vi "探头模板-12-网络版.vi"(11 "探头序号":T12(ring) caption="探头地址") -> ()   [LabVIEW 2017]
uses:
  <vilib>/Utility/miscctls.llb/LVPoint32TypeDef.ctl
  <vilib>/Utility/miscctls.llb/LVPositionTypeDef.ctl
  472b0359-2eb9-43bd-80a0-de906e95224b.vi
panel:
  out "初始尺寸":T1
  out "报警方式a":T2
  out "探头状态a":T3
  in  "报警方式[]":string[](array[string])
  out "累积":string="累积剂量/限值："
  in  "鼠标坐标":T4 caption="坐标"
  out "计算时间":dbl
  in  "坐标映射信号":bool=TRUE
  in  "探头属性":T5={"探头地址与信息"={"网络地址"="", "名称"="", "备注"="", "累积剂量"=0.0, "累积限值"=0.0, "硬件剂量率限值"=enum."一级限值", "剂量率限值1"=0.0, "剂量率限值2"=0.0, "报警方式"=enum."常报警"}, "测量值"={"时间"=timestamp(3554955153.6246996 s since 1904-01-01), "数值"=0.0}, "限值"={"限值1"=0.0, "限值2"=0.0, "探头限值"=enum."一级限值"}, "探头状态"=enum."正常", "累积记录"={"起始时间"=timestamp(0 s since 1904-01-01), "结束时间"=timestamp(0 s since 1904-01-01), "累积剂量"=0.0}, "报警方式"={"报警方式"=enum."常报警", "延迟计时"=0, "报警中？"=FALSE}}
  in  "停止":bool=TRUE
  out "探头地址":T12(ring)
  out "探头状态":enum16{"正常", "离线", "禁用", "一级报警", "二级报警", "累积报警"}(ring)=enum."一级报警"
  out "探头信息":string
  out "测量值":dbl format="%.2g"
  out "单位":enum16{"μ", "m"}(ring)
  out "限值1":string="一级限值："
  out "限值2":string="二级限值："
  out "数值":string="一级限值："
  in  "XY图":cluster{timestamp[], dbl[]}[](graph)
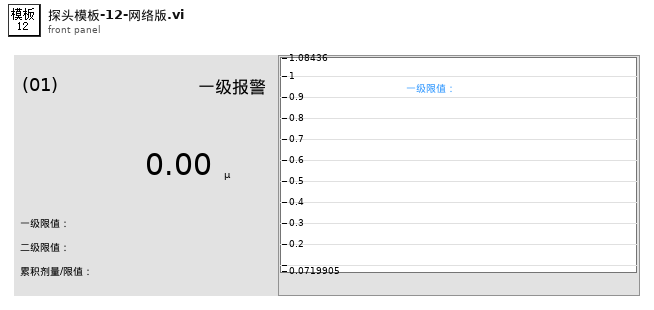
[diagram p1: front panel]
types:
  T1 = typedef "簇-界面模板初始字号.ctl" = cluster{"边界:区域高度":u32, "最大字号":cluster{"限值信息":u32, "测量值":u32, "序号":u32, "名称":u32, "单位":u32, "状态":u32, "悬浮框":u32}}
  T2 = typedef "报警方式选择.ctl" = enum16{"常报警", "自动静音", "手动静音"}
  T3 = typedef "探头状态.ctl" = enum16{"正常", "离线", "禁用", "一级报警", "二级报警", "累积报警"}
  T4 = typedef "LVPoint32TypeDef.ctl" = cluster{"Horizontal":i32, "Vertical":i32}
  T5 = typedef "探头属性.ctl" = cluster{"探头地址与信息":T6, "测量值":T8, "限值":T9, "探头状态":T3, "累积记录":T10, "报警方式":T11}
  T6 = typedef "探测器信息.ctl" = cluster{"网络地址":string, "名称":string, "备注":string, "累积剂量":dbl, "累积限值":dbl, "硬件剂量率限值":T7, "剂量率限值1":dbl, "剂量率限值2":dbl, "报警方式":T2}
  T7 = typedef "探头剂量率限值选择.ctl" = enum16{"一级限值", "二级限值"}
  T8 = typedef "测量值.ctl" = cluster{"时间":timestamp, "数值":dbl}
  T9 = typedef "剂量率限值.ctl" = cluster{"限值1":dbl, "限值2":dbl, "探头限值":T7}
  T10 = typedef "单条累积记录.ctl" = cluster{"起始时间":timestamp, "结束时间":timestamp, "累积剂量":dbl}
  T11 = typedef "报警方式.ctl" = cluster{"报警方式":T2, "延迟计时":u16, "报警中？":bool}
  T12 = enum16{"(01)", "(02)", "(03)", "(04)", "(05)", "(06)", "(07)", "(08)", "(09)", "(10)", "(11)", "(12)", "(13)", "(14)", "(15)", "(16)", "(17)", "(18)", "(19)", "(20)", "(21)", "(22)", "(23)", "(24)", "(25)", "(26)", "(27)", "(28)", "(29)", "(30)", "(31)", "(32)", "(33)", "(34)", "(35)"}
  T13 = cluster{"限值信息":u32, "测量值":u32, "序号":u32, "名称":u32, "单位":u32, "状态":u32, "悬浮框":u32}
  T14 = typedef "LVPositionTypeDef.ctl" = cluster{"Left":i32, "Top":i32}
  T15 = cluster{"原始尺寸":cluster{"所在窗格高度":u32, "字号":u32}, "new所在窗格高度":u32}
  T16 = enum16{"No Scaling", "Scale All Objects", "Scale Single Object"}
  T17 = typedef "LVBoundsTypeDef.ctl" = cluster{"Width":u32, "Height":u32}
  T18 = enum8{"Enabled", "Disabled", "Disabled and Grayed Out"}
  T19 = typedef "LVRectTypeDef.ctl" = cluster{"Left":i16, "Top":i16, "Right":i16, "Bottom":i16}
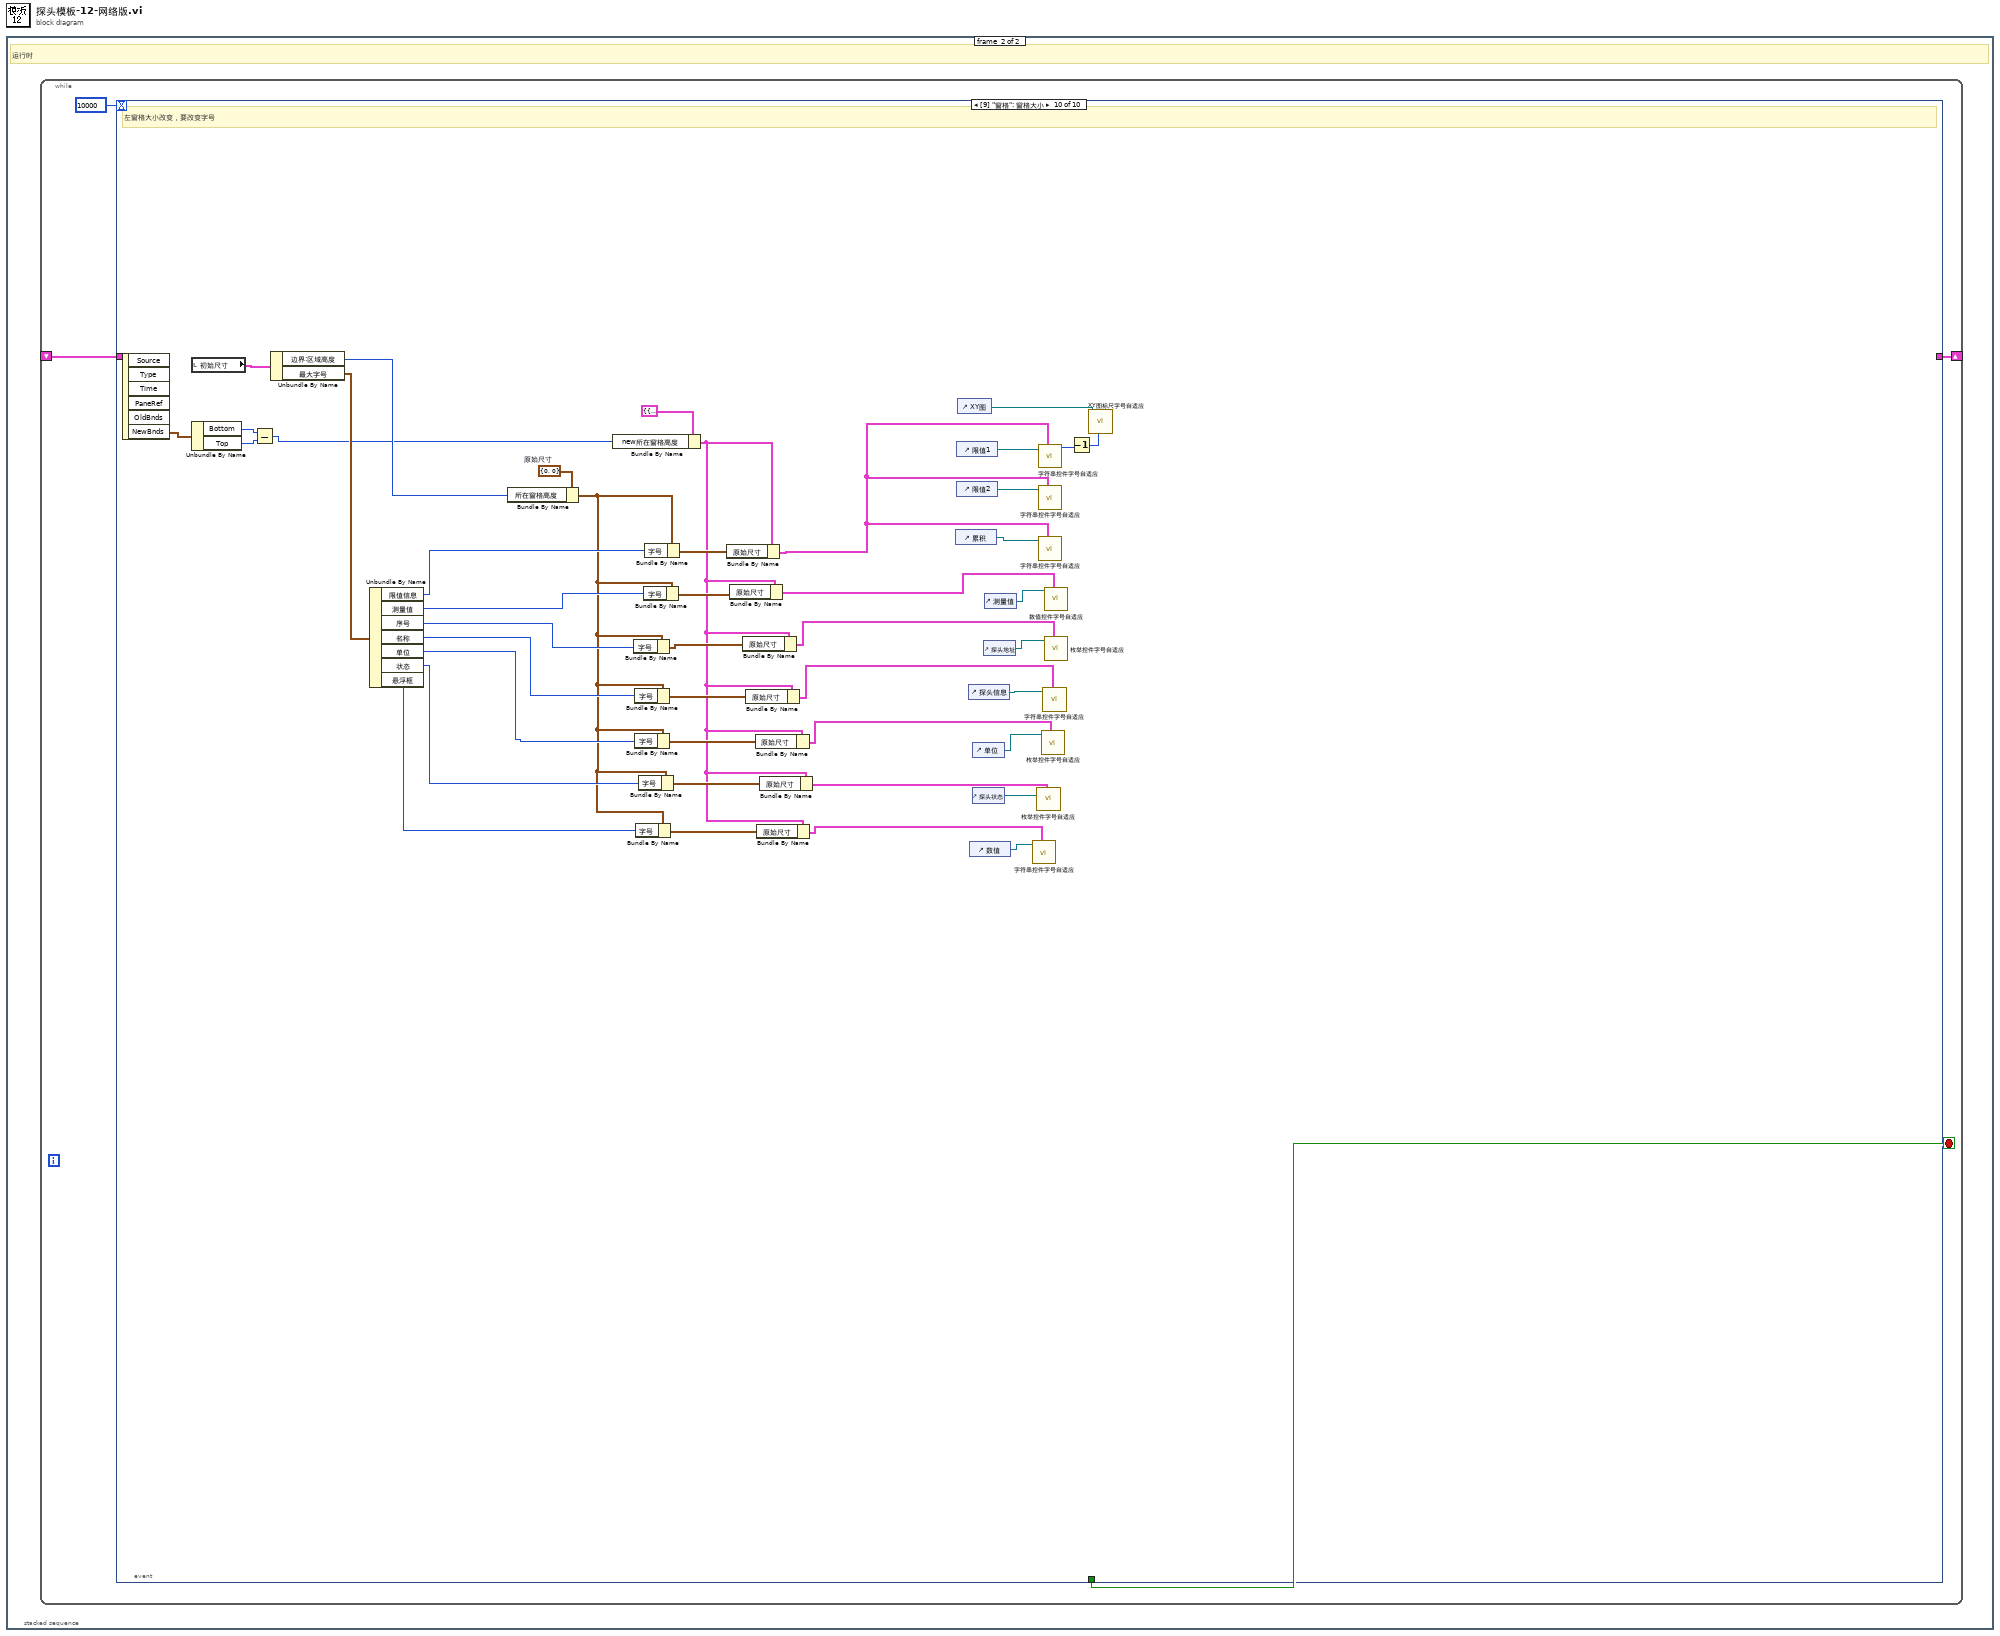
[diagram p0: block diagram]
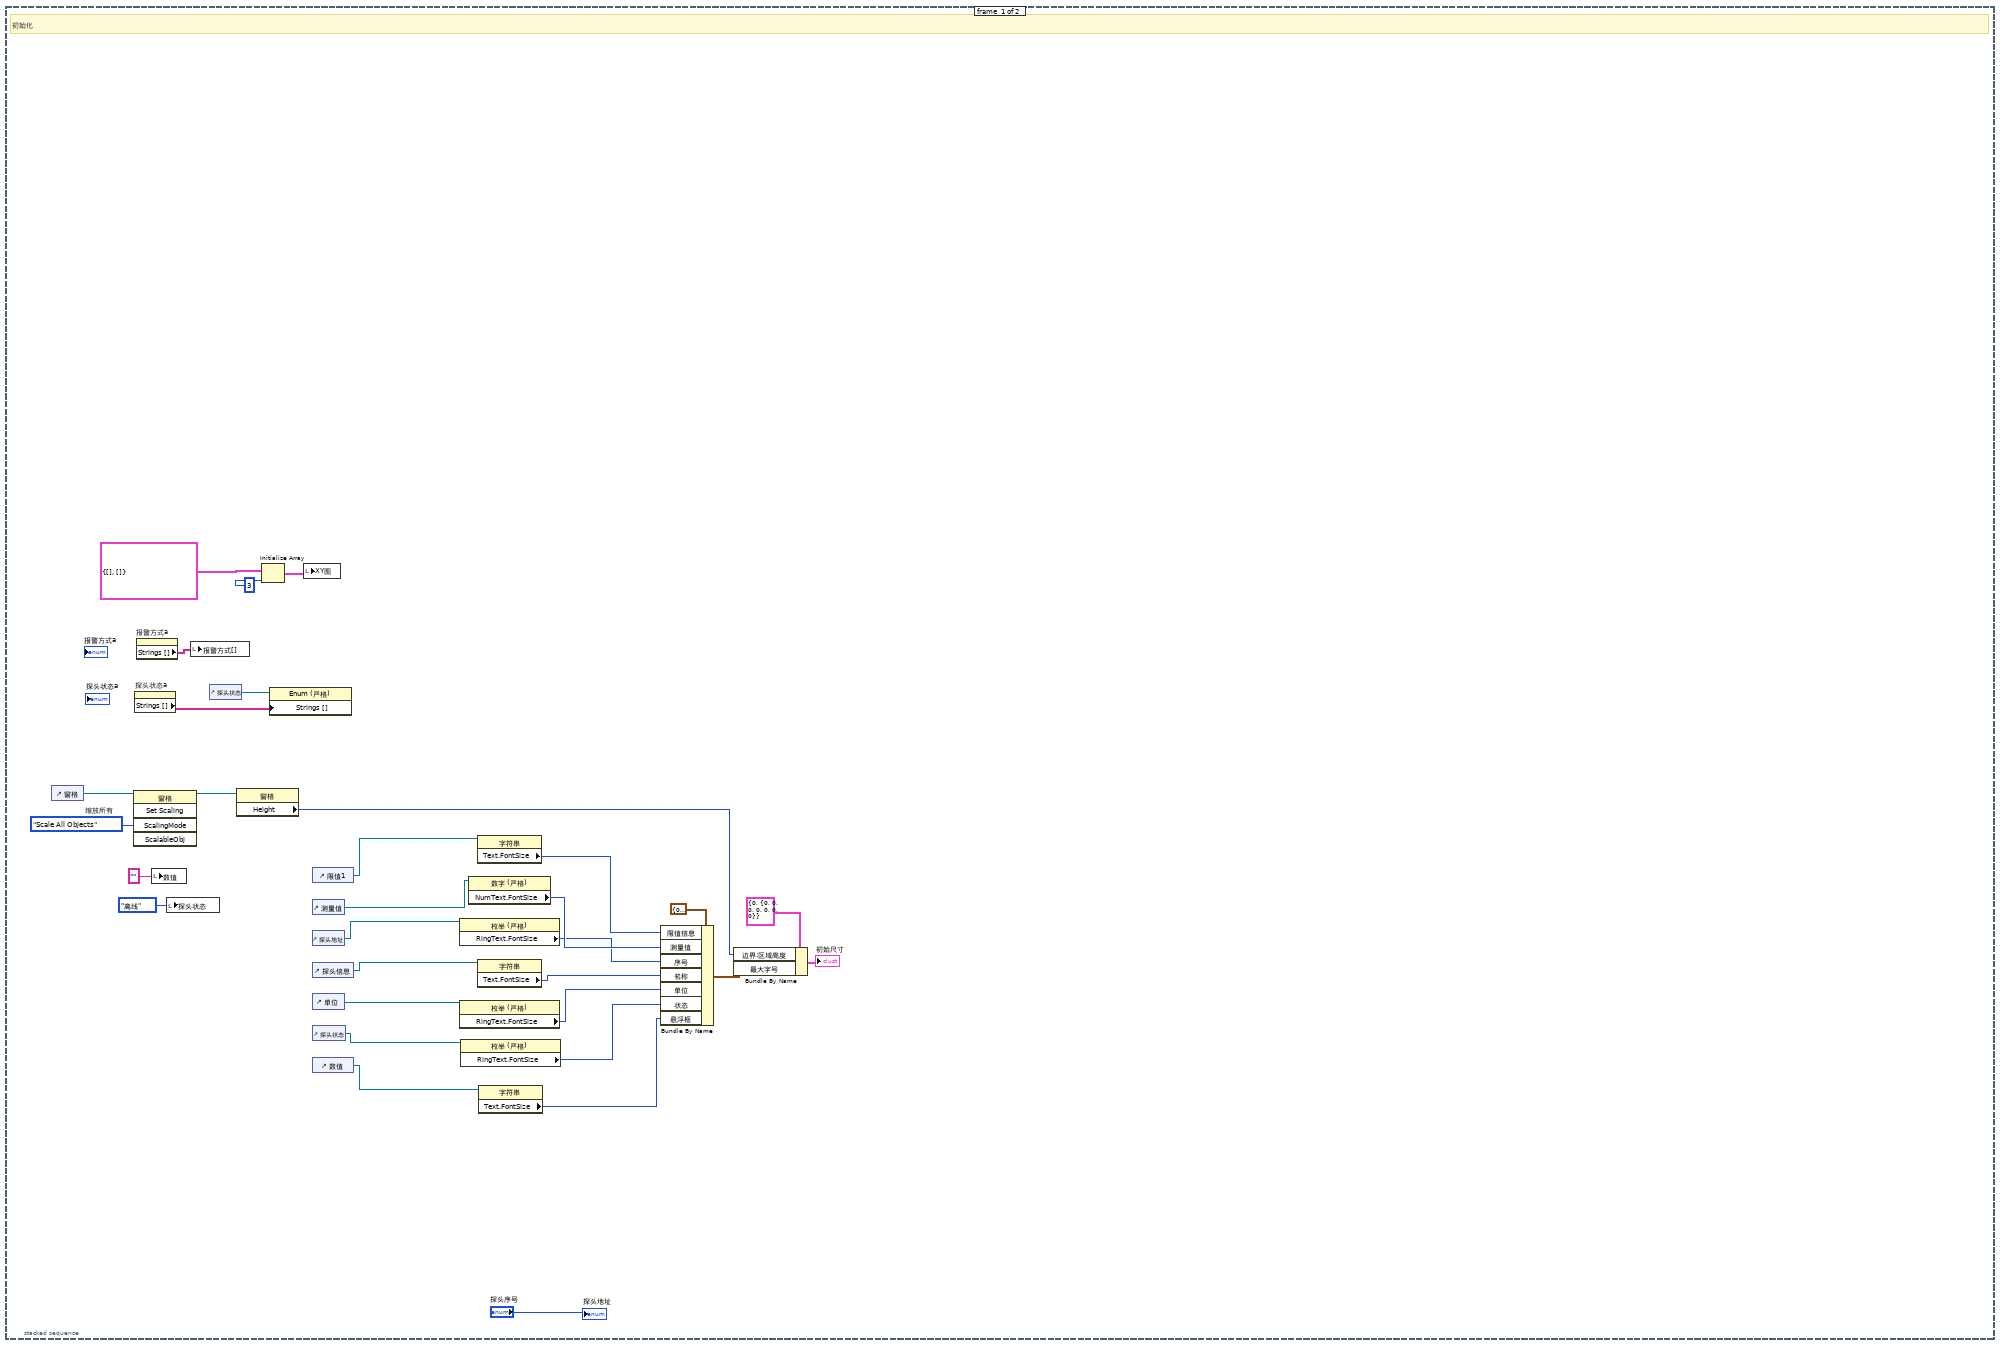
[diagram p2: hidden frame]
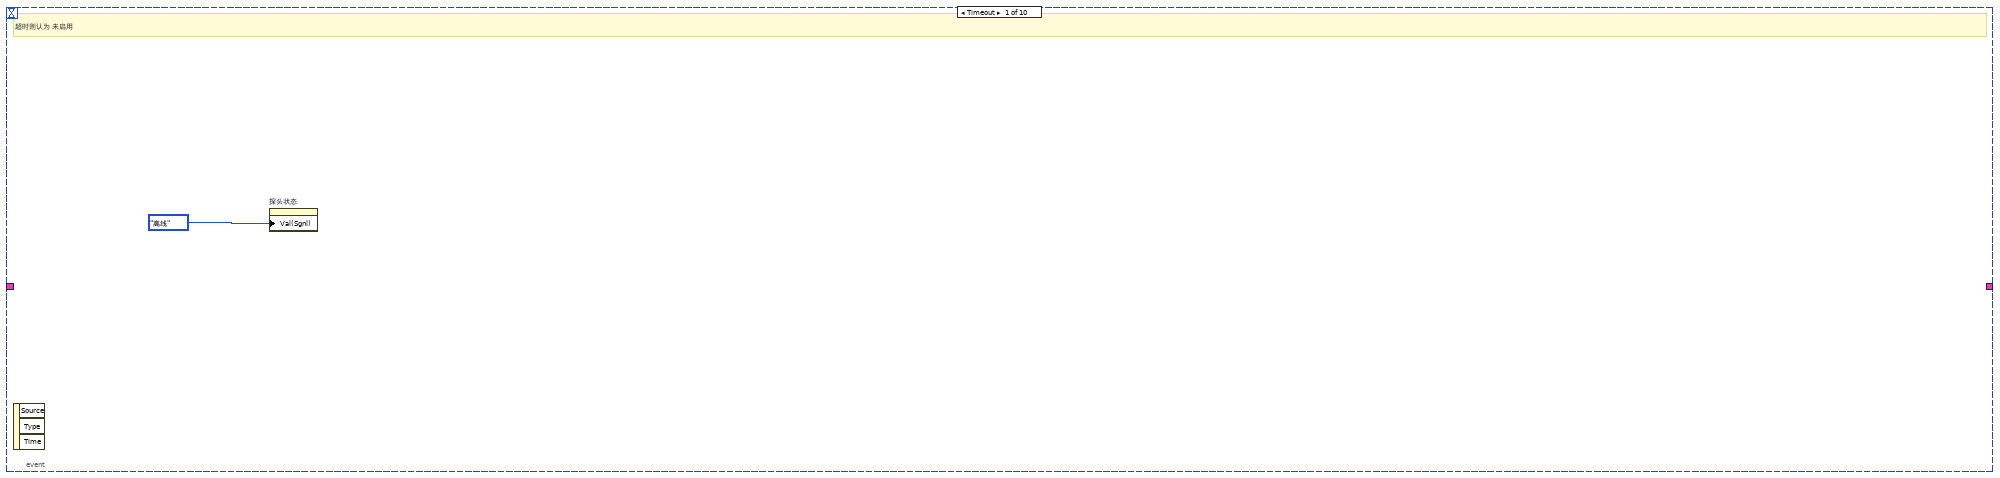
[diagram p3: hidden frame]
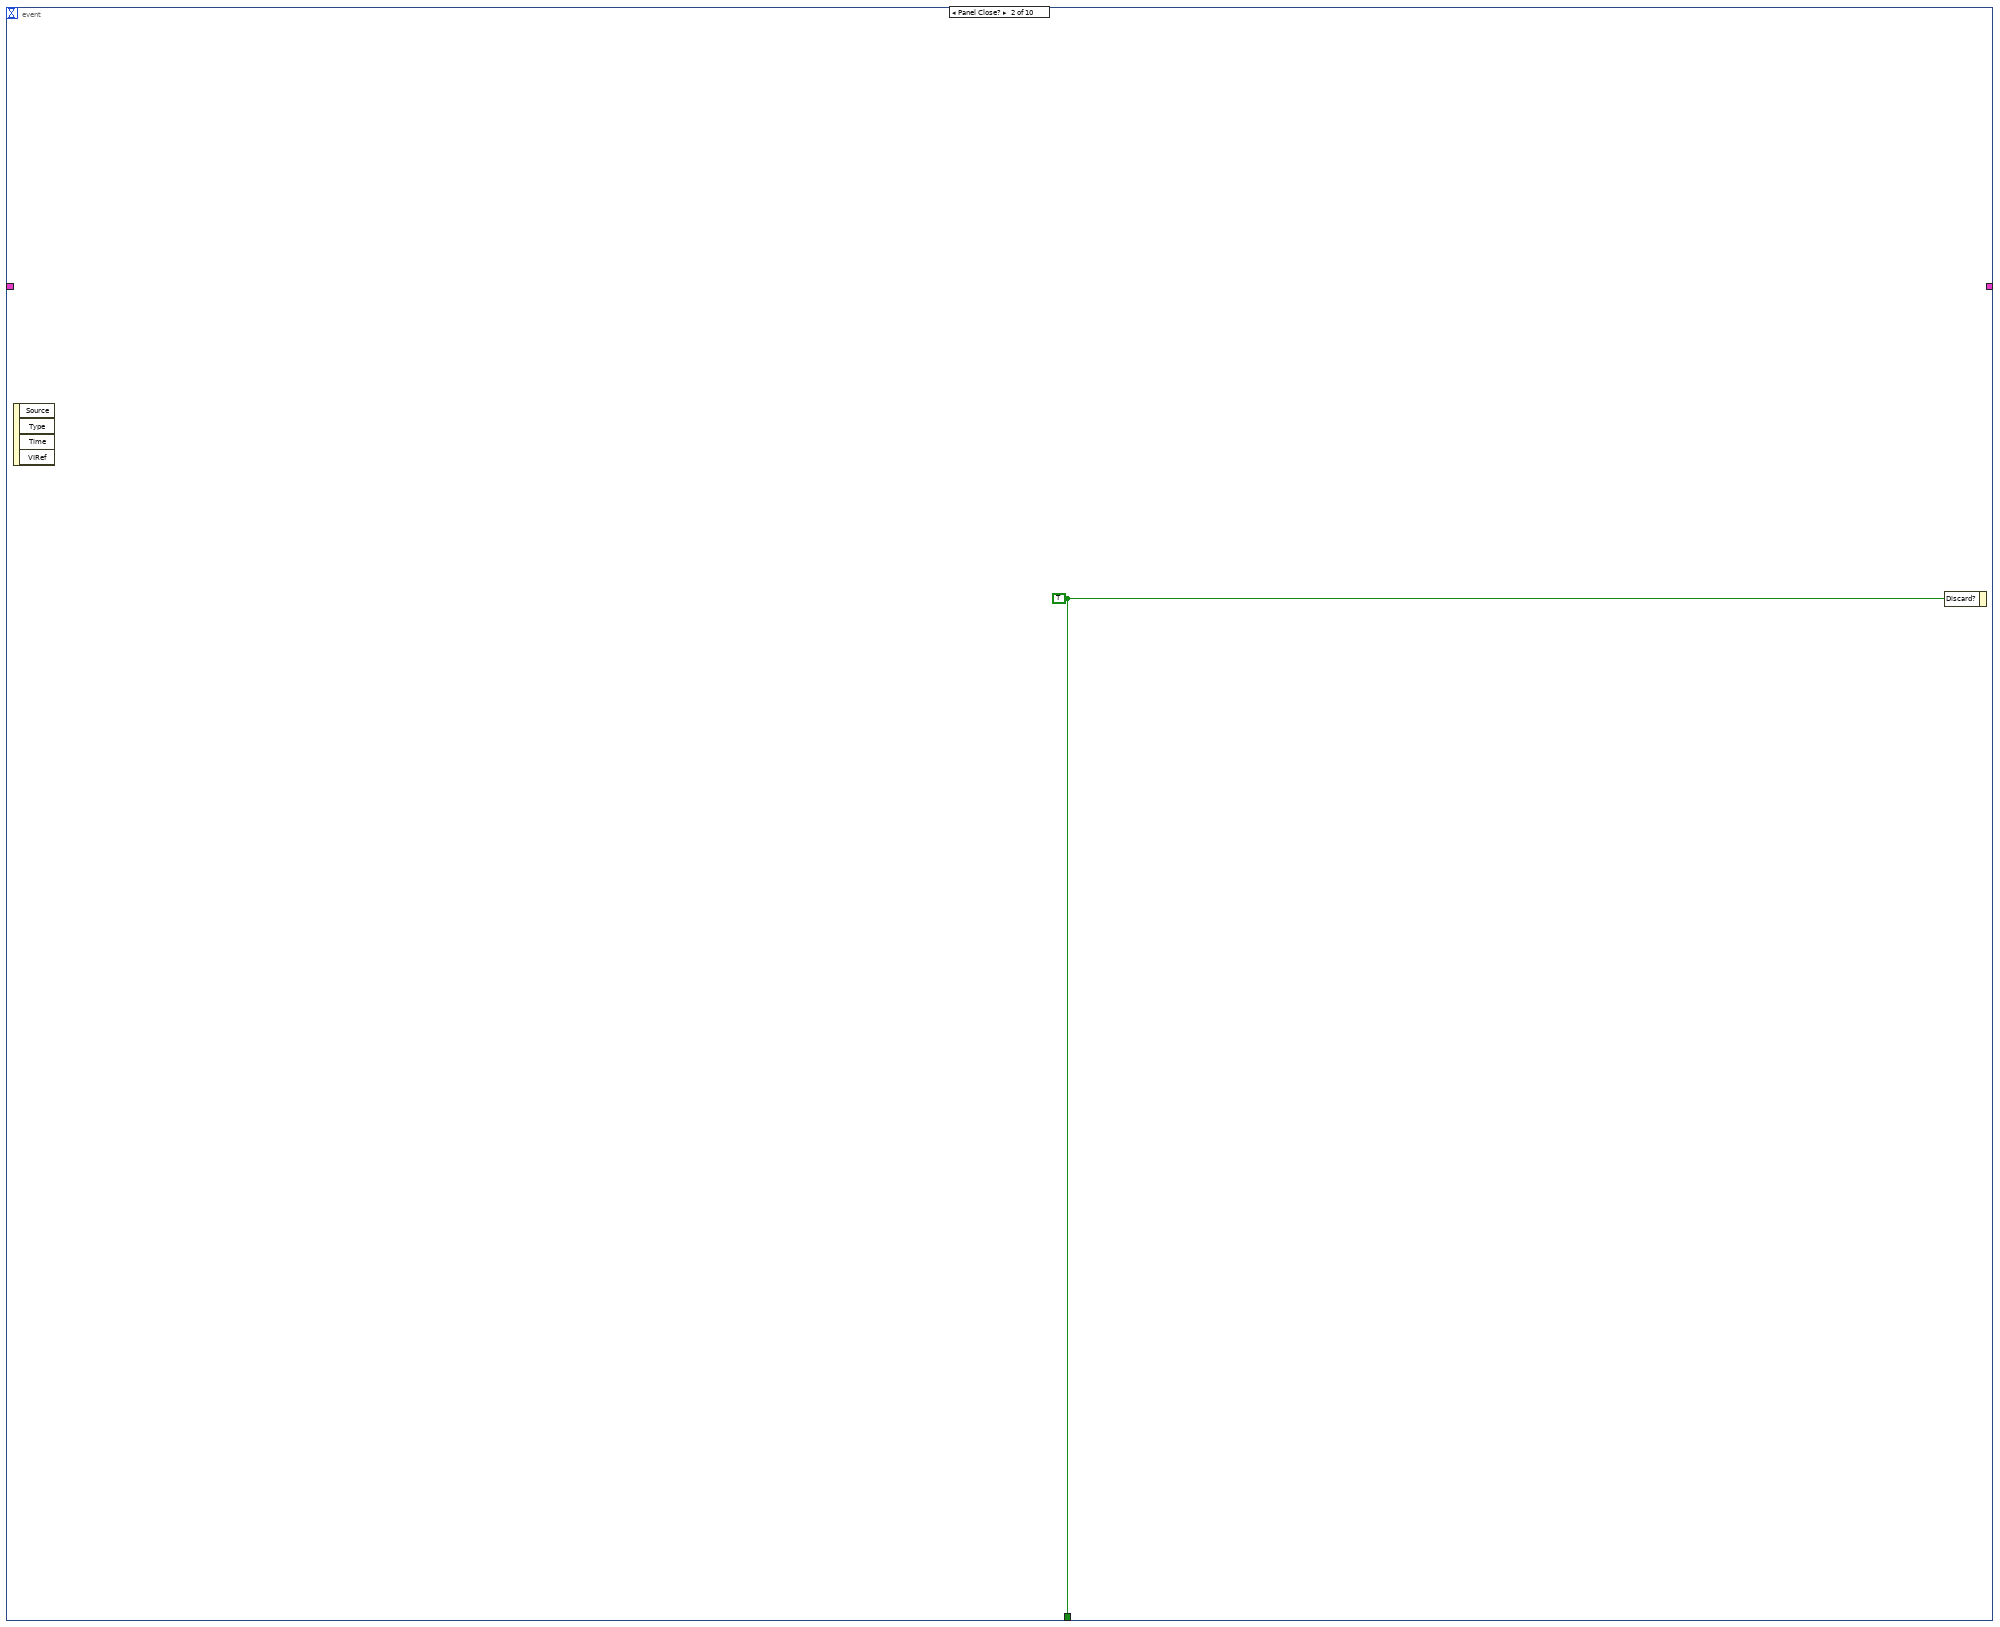
[diagram p4: hidden frame]
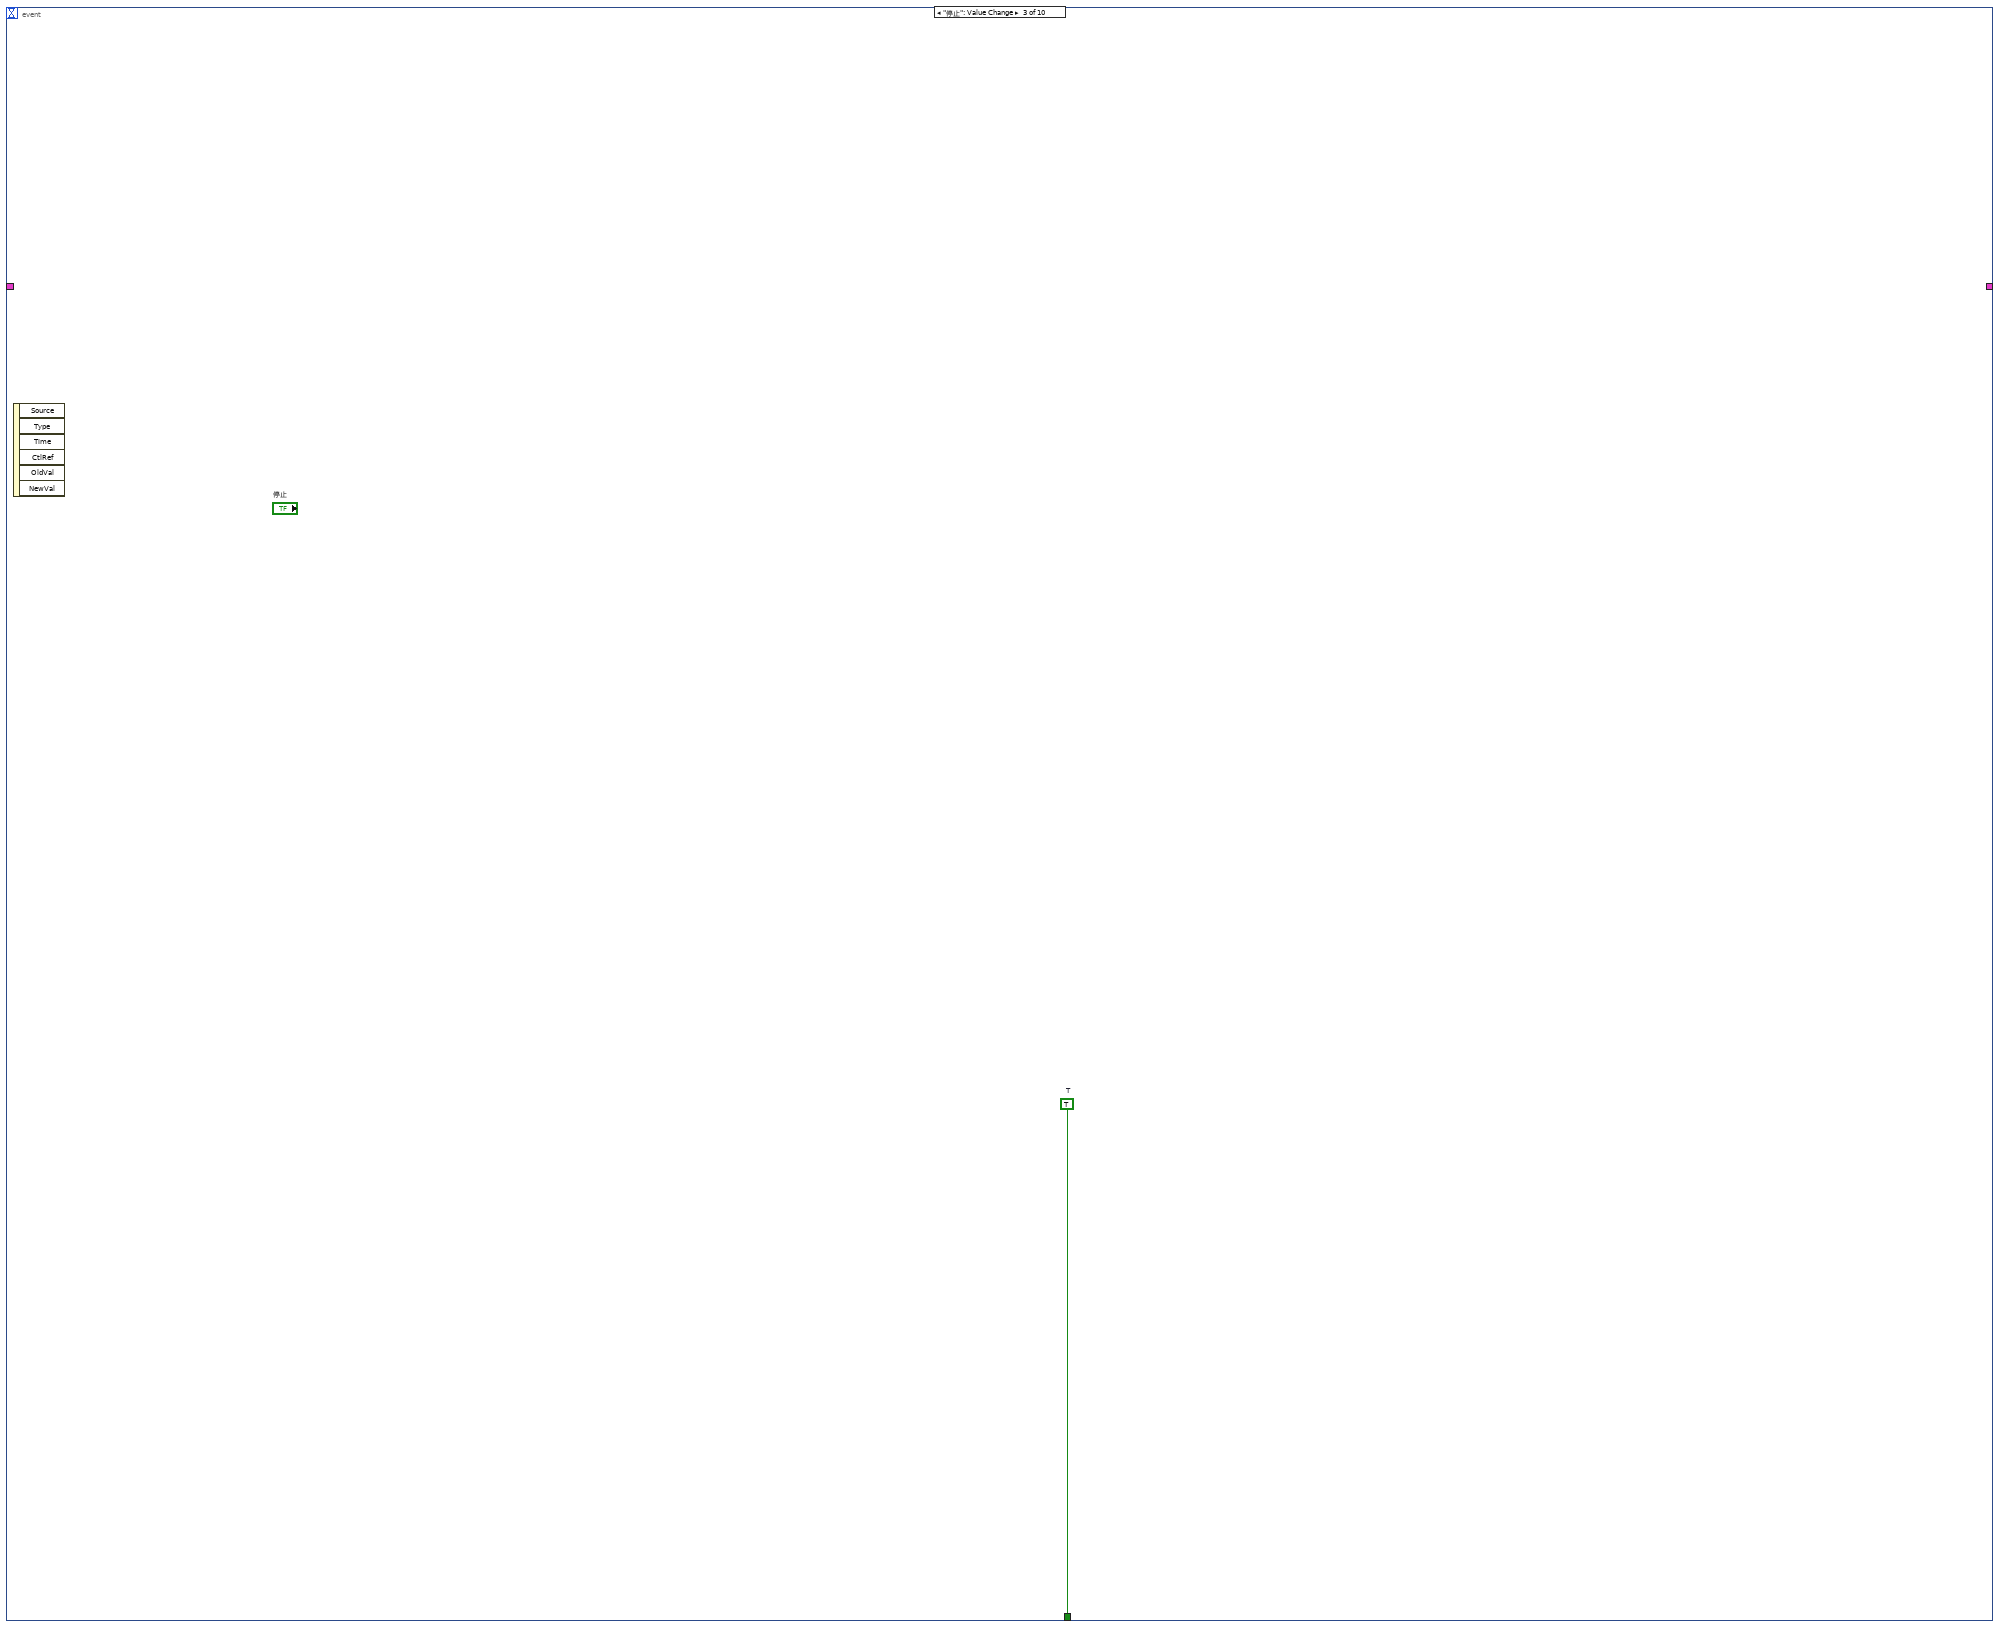
[diagram p5: hidden frame]
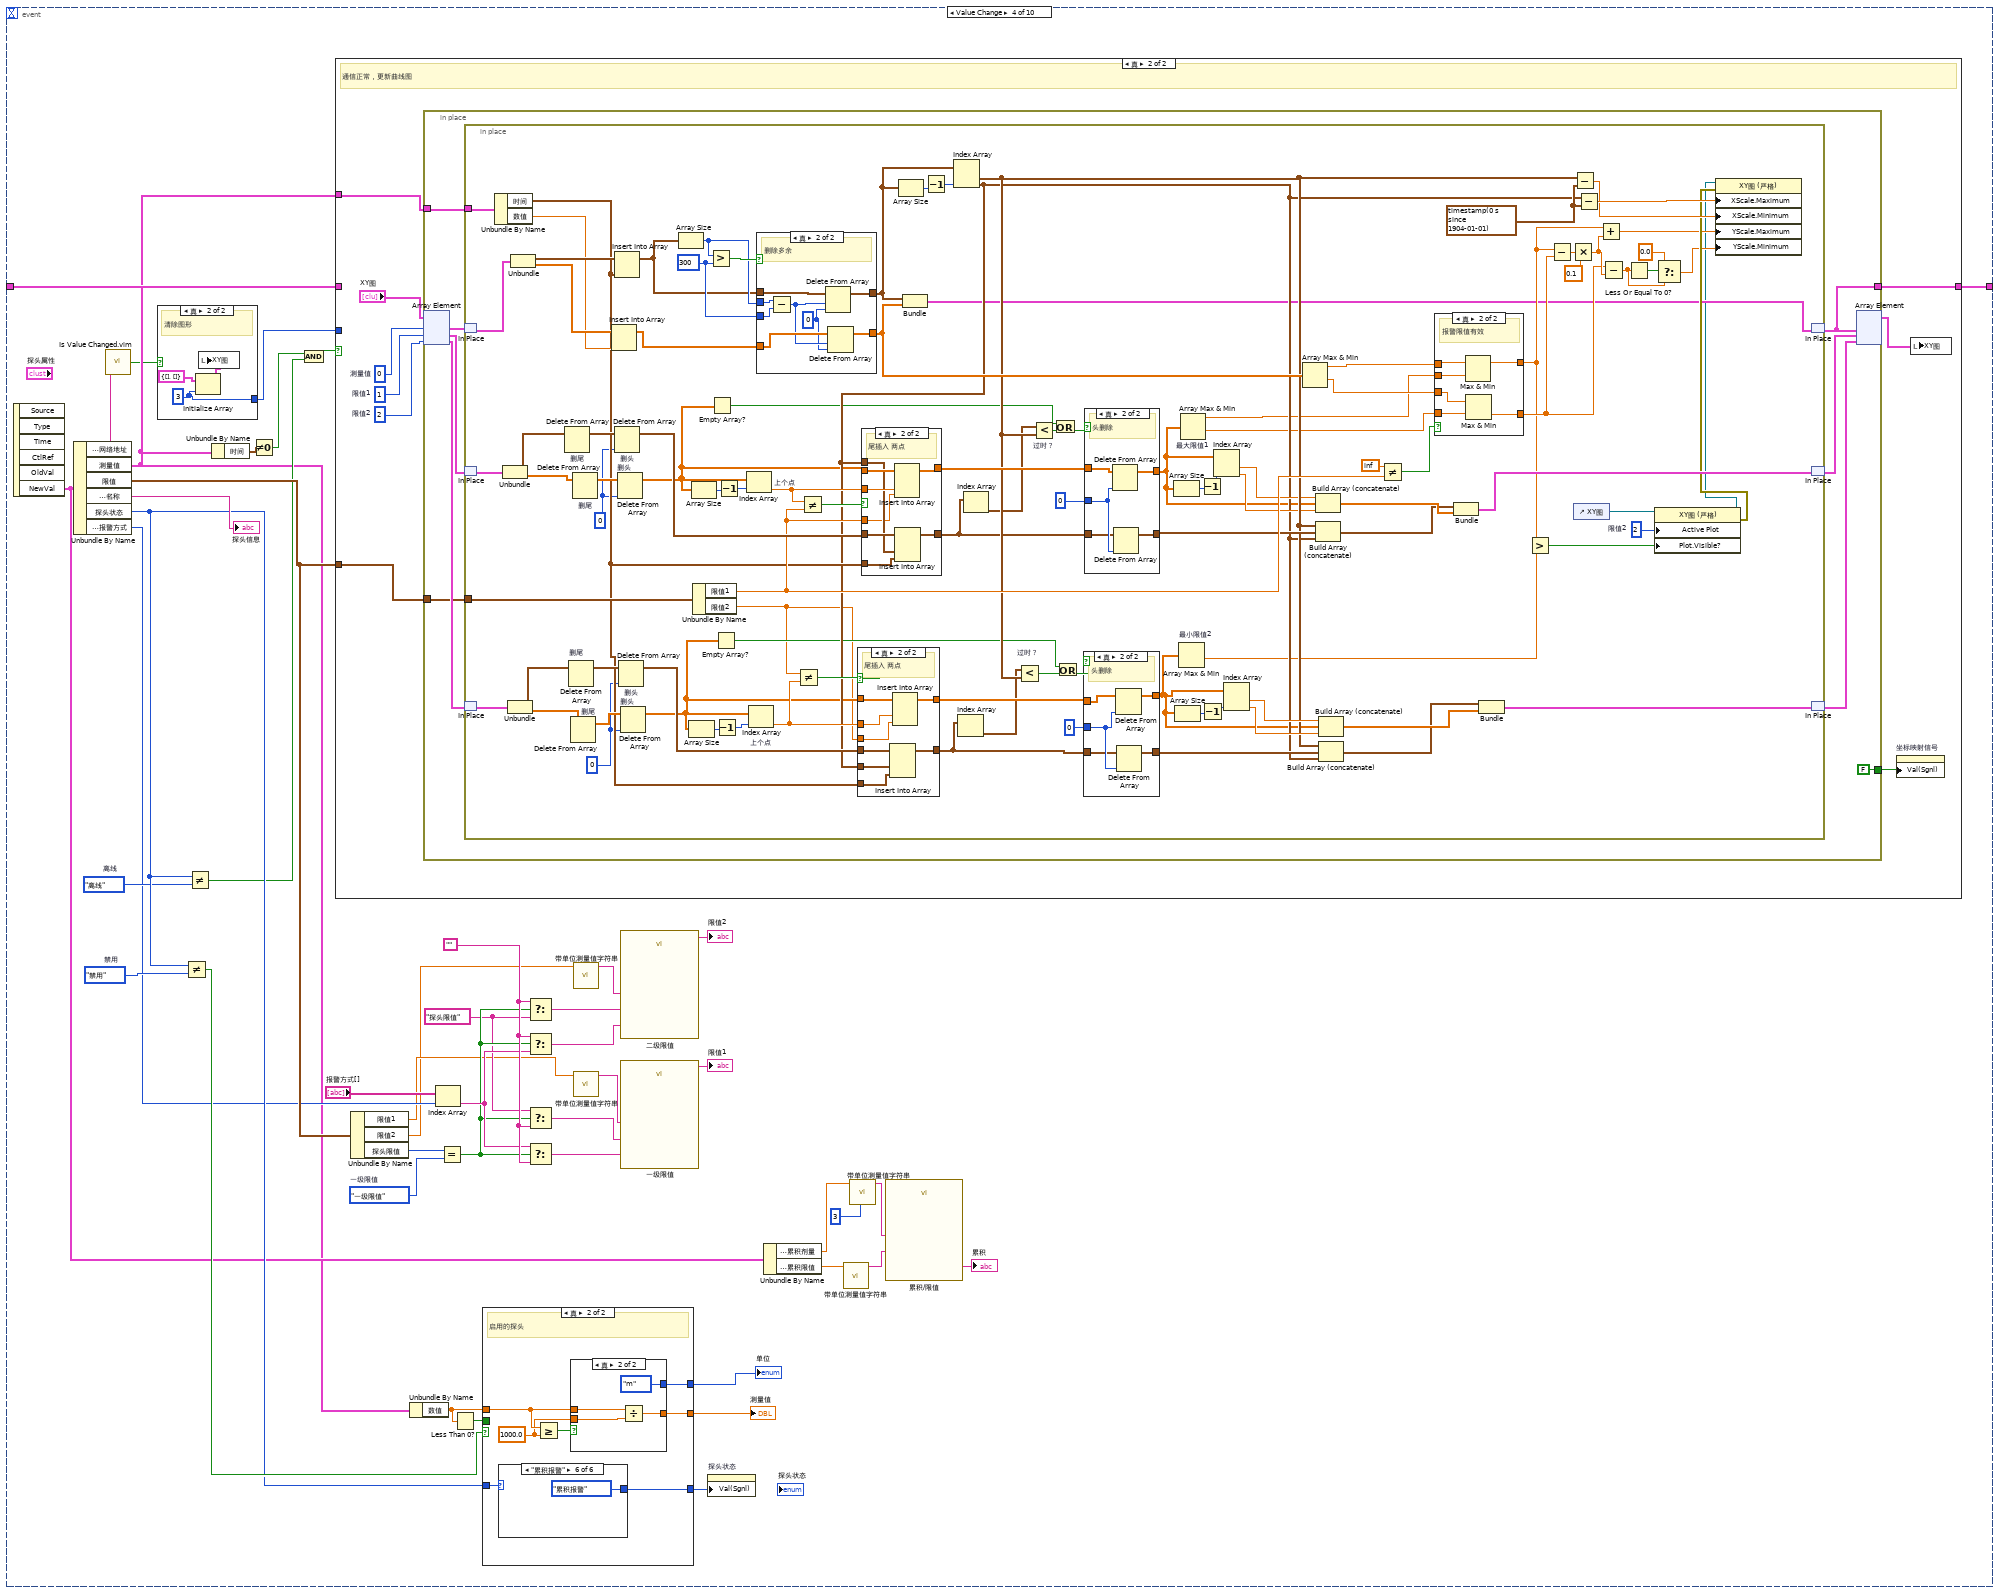
[diagram p6: hidden frame]
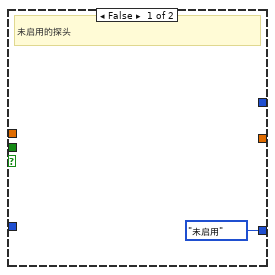
[diagram p15: hidden frame]
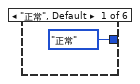
[diagram p16: hidden frame]
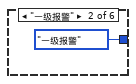
[diagram p17: hidden frame]
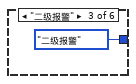
[diagram p18: hidden frame]
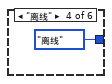
[diagram p19: hidden frame]
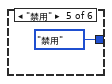
[diagram p20: hidden frame]
diagram:
  n1 = stacked-sequence {
    frame #0 {
      w24 = T16."Scale All Objects"  # 缩放所有
      # "初始化"
      n2 = control-ref of="窗格"() -> (w23:refnum<vi>)
      n3 = invoke class="窗格" method="Set Scaling"(reference=w23, "ScalingMode"=w24) -> (reference out=w20:refnum<vi>)  [unwired: 3 in, 4 out]
      n4 = property on="探头状态a" class="Enum (严格)"() -> ("Strings []"=w22:string[])  [unwired: 2 in, 2 out]
      n5 = property on="报警方式a" class="Enum (严格)"() -> ("Strings []"=w25:string[])  [unwired: 2 in, 2 out]
      n6 = local write "数值"("" ("数值")) -> ()
      n7 = local write "探头状态"(探头状态."离线" ("探头状态")) -> ()
      n8 = local write "报警方式[]"(w25) -> ()
      n9 = control-ref of="探头状态"() -> (w26:refnum<vi>)
      n10 = property class="窗格"(reference=w20) -> ("Height"=w1:u32)  [unwired: 1 in, 2 out]
      n11 = Initialize Array(cluster{timestamp[], dbl[]} {[], []}, 3 ("维数大小")) -> (w21:cluster{timestamp[], dbl[]}[])
      n12 = property on="属性节点" class="Enum (严格)"(reference=w26, "Strings []"=w22) -> ()  [unwired: 1 in, 2 out]
      n13 = local write "XY图"(w21) -> ()
      n14 = control-ref of="限值1"() -> (w15:refnum<vi>)
      n15 = control-ref of="测量值"() -> (w14:refnum<vi>)
      n16 = control-ref of="探头地址"() -> (w13:refnum<vi>)
      n17 = control-ref of="探头信息"() -> (w12:refnum<vi>)
      n18 = control-ref of="单位"() -> (w11:refnum<vi>)
      n19 = control-ref of="数值"() -> (w9:refnum<vi>)
      n20 = control-ref of="探头状态"() -> (w10:refnum<vi>)
      n21 = property class="枚举 (严格)"(reference=w13) -> ("RingText.FontSize"=w6:u32)  [unwired: 1 in, 2 out]
      n22 = property class="枚举 (严格)"(reference=w11) -> ("RingText.FontSize"=w4:u32)  [unwired: 1 in, 2 out]
      n23 = property class="枚举 (严格)"(reference=w10) -> ("RingText.FontSize"=w3:u32)  [unwired: 1 in, 2 out]
      n24 = property class="数字 (严格)"(reference=w14) -> ("NumText.FontSize"=w7:u32)  [unwired: 1 in, 2 out]
      n25 = property class="字符串"(reference=w15) -> ("Text.FontSize"=w8:u32)  [unwired: 1 in, 2 out]
      n26 = property class="字符串"(reference=w12) -> ("Text.FontSize"=w5:u32)  [unwired: 1 in, 2 out]
      n27 = property class="字符串"(reference=w9) -> ("Text.FontSize"=w2:u32)  [unwired: 1 in, 2 out]
      n28 = Bundle By Name(cluster=T13 {"限值信息"=0, "测量值"=0, "序号"=0, "名称"=0, "单位"=0, "状态"=0, "悬浮框"=0} ("最大字号"), "限值信息"=w8, "测量值"=w7, "序号"=w6, "名称"=w5, "单位"=w4, "状态"=w3, "悬浮框"=w2) -> (w19:T13)
      n29 = Bundle By Name(cluster=T1 {"边界:区域高度"=0, "最大字号"={"限值信息"=0, "测量值"=0, "序号"=0, "名称"=0, "单位"=0, "状态"=0, "悬浮框"=0}} ("输出簇"), "边界:区域高度"=w1, "最大字号"=w19) -> (→"初始尺寸":T1)
      "探头地址" <- "探头序号"
    }
    frame #1 {
      # "运行时"
      n30 = while {
        shift-right: [w34] -> _
        shift-left: _ -> [w33]
        stop <- w35 stop-if-true
        n31 = event shown="[9] \"窗格\": 窗格大小" {
          selector: _ -> [_ _ _ _ _ _ _ _ _ _]
          dyn-events: _ -> [_ _ _ _ _ _ _ _ _ _]
          timeout: 10000 -> [_ _ _ _ _ _ _ _ _ _]
          tunnel: [_ w37 w38 _ _ _ _ _ _ _] -> w35
          tunnel: [_ _ _ w72 w281 w283 w285 w290 w351 _] -> w34
          tunnel: w33 -> [_ _ _ w71 w281 w283 w285 w290 w351 _]
          event Timeout {
            # "超时则认为 未启用"
            n32 = event-data() -> ()  [unwired: 1 in, 3 out]
            n33 = property on="探头状态" class="Enum (严格)"("Val(Sgnl)"=探头状态."离线" ("值(信号)")) -> ()  [unwired: 2 in, 2 out]
          }
          event Panel Close? {
            w37 = TRUE ("放弃？")
            n34 = event-data() -> ()  [unwired: 1 in, 4 out]
            n35 = event-data("Discard?"=w37) -> ()  [unwired: 1 in, 1 out]
          }
          event "停止": Value Change {
            w38 = TRUE  # T
            n36 = event-data() -> ()  [unwired: 1 in, 6 out]
          }
          event Value Change {
            w70 = ""
            w67 = "探头限值" ("F-格式字符串")
            w66 = 探头剂量率限值选择."一级限值"  # 一级限值
            w74 = 探头状态."离线"  # 离线
            w79 = 探头状态."禁用"  # 禁用
            n37 = event-data() -> ("NewVal"=w63:T5)  [unwired: 1 in, 5 out]
            n38 = Unbundle By Name(w63) -> ("探头地址与信息.网络地址"=w41:string, "测量值"=w44:T8, "限值"=w78:T9, "探头地址与信息.名称"=→"探头信息":string, "探头状态"=w75:T3, "探头地址与信息.报警方式"=w64:T2)
            n39 = call "Is Value Changed.vim"("value"=w41) -> ("changed or first call?"=w40:bool)
            n40 = case shown="真" w40 {
              tunnel: [_ w85] -> w39
              frame False {
              }
              frame True {
                w85 = 3 ("维数大小")
                # "清除图形"
                n41 = Initialize Array(cluster{timestamp[], dbl[]} {[], []}, w85) -> (w86:cluster{timestamp[], dbl[]}[])
                n42 = local write "XY图"(w86) -> ()
              }
            }
            n43 = Not Equal?(x=w75, y=w79) -> (x != y?=w76:bool)
            n44 = Not Equal?(x=w75, y=w74) -> (x != y?=w73:bool)
            n45 = Unbundle By Name(w44) -> ("时间"=w43:timestamp)
            n46 = Not Equal To 0?(x=w43) -> (x != 0?=w42:bool)
            n47 = And(x=w42, y=w73) -> (x .and. y?=w45:bool)
            n48 = case shown="真" w45 {
              tunnel: w44 -> [_ w97]
              tunnel: w78 -> [_ w92]
              tunnel: [w88 w90] -> w72
              tunnel: w71 -> [w88 _]
              tunnel: w39 -> [_ _]
              frame False {
                # "离线，不更新"
              }
              frame True {
                w93 = 2  # 限值2
                w94 = 1  # 限值1
                w95 = 0  # 测量值
                # "通信正常，更新曲线图"
                n49 = in-place {
                  in-place-border: w97 -> [w106]
                  in-place-border: w92 -> [w102]
                  in-place-border: [w99] -> w90
                  in-place-border: [FALSE ("值(信号)")] -> w89
                  n50 = in-place-array #1("XY图", w95, w94, w93) -> (w105:cluster{timestamp[], dbl[]}, w103:cluster{timestamp[], dbl[]}, w104:cluster{timestamp[], dbl[]})
                  n51 = in-place {
                    in-place-border: w106 -> [w202]
                    in-place-border: w102 -> [w196]
                    w132 = 0 ("索引")
                    w133 = 0 ("索引")
                    w194 = u32 2  # 限值2
                    w203 = 300 ("y")
                    w208 = timestamp(0 s since 1904-01-01)
                    n52 = in-place-match #2(w105) -> (w197:cluster{timestamp[], dbl[]})
                    n53 = in-place-match #3(w103) -> (w162:cluster{timestamp[], dbl[]})
                    n54 = in-place-match #4(w104) -> (w143:cluster{timestamp[], dbl[]})
                    n55 = Unbundle By Name(w202) -> ("时间"=w142:timestamp, "数值"=w193:dbl)
                    n56 = Unbundle(w162) -> (w166:timestamp[], w165:dbl[])
                    n57 = Unbundle(w143) -> (w147:timestamp[], w146:dbl[])
                    n58 = Unbundle(w197) -> (w201:timestamp[], w200:dbl[])
                    n59 = Delete From Array "删尾"(array=w166) -> (array with subset deleted=w167:timestamp[])  [unwired: 2 in, 1 out]
                    n60 = Delete From Array "删尾"(array=w147) -> (array with subset deleted=w148:timestamp[])  [unwired: 2 in, 1 out]
                    n61 = Delete From Array "删尾"(array=w146) -> (array with subset deleted=w145:dbl[])  [unwired: 2 in, 1 out]
                    n62 = Delete From Array "删尾"(array=w165) -> (array with subset deleted=w164:dbl[])  [unwired: 2 in, 1 out]
                    n63 = Insert Into Array(array=w200, new element=w193) -> (w198:dbl[])  [unwired: 1 in]
                    n64 = Insert Into Array(array=w201, new element=w142) -> (w199:timestamp[])  [unwired: 1 in]
                    n65 = Delete From Array "删头"(array=w167, index=w133) -> (array with subset deleted=w170:timestamp[])  [unwired: 1 in, 1 out]
                    n66 = Delete From Array "删头"(array=w164, index=w133) -> (array with subset deleted=w121:dbl[])  [unwired: 1 in, 1 out]
                    n67 = Delete From Array "删头"(array=w148, index=w132) -> (array with subset deleted=w152:timestamp[])  [unwired: 1 in, 1 out]
                    n68 = Delete From Array "删头"(array=w145, index=w132) -> (array with subset deleted=w120:dbl[])  [unwired: 1 in, 1 out]
                    n69 = Array Size(array=w199) -> (size(s)=w204:i32)
                    n70 = Array Size(array=w120) -> (size(s)=w149:i32)
                    n71 = Array Size(array=w121) -> (size(s)=w163:i32)
                    n72 = Unbundle By Name(w196) -> ("限值1"=w161:dbl, "限值2"=w115:dbl)
                    n73 = Greater?(x=w204, y=w203) -> (0:w205:bool)
                    n74 = Empty Array?(array=w121) -> (empty?=w119:bool)
                    n75 = Empty Array?(array=w120) -> (empty?=w118:bool)
                    n76 = Decrement(x=w149) -> (x-1=w150:i32)
                    n77 = Decrement(x=w163) -> (x-1=w168:i32)
                    n78 = Index Array "上个点"(array=w121, index=w168) -> (element=w131:dbl)
                    n79 = Index Array "上个点"(array=w120, index=w150) -> (element=w130:dbl)
                    n80 = case shown="真" w205 {
                      tunnel: w199 -> [w252 w260]
                      tunnel: w204 -> [_ w259]
                      tunnel: w203 -> [_ w258]
                      tunnel: [w252 w257] -> w192
                      tunnel: w198 -> [w251 w256]
                      tunnel: [w251 w253] -> w188
                      frame False {
                      }
                      frame True {
                        w254 = 0 ("索引")
                        # "删除多余"
                        n81 = Subtract(x=w259, y=w258) -> (x-y=w255:i32)
                        n82 = Delete From Array(array=w260, length=w255, index=w254) -> (array with subset deleted=w257:timestamp[])  [unwired: 1 out]
                        n83 = Delete From Array(array=w256, length=w255, index=w254) -> (array with subset deleted=w253:dbl[])  [unwired: 1 out]
                      }
                    }
                    n84 = Not Equal?(x=w115, y=w130) -> (x != y?=w144:bool)
                    n85 = Not Equal?(x=w131, y=w161) -> (x != y?=w134:bool)
                    n86 = Array Size(array=w192) -> (size(s)=w191:i32)
                    n87 = Bundle(w192, w188) -> (w109:cluster{timestamp[], dbl[]})  [unwired: 1 in]
                    n88 = Decrement(x=w191) -> (x-1=w190:i32)
                    n89 = Index Array(array=w192, index #2=w190) -> (element #1=w139:timestamp, element #2=w129:timestamp)  [unwired: 1 in]
                    n90 = case shown="真" w144 {
                      tunnel: [w217 w219] -> w128
                      tunnel: w120 -> [w217 w225]
                      tunnel: w115 -> [_ w218]
                      tunnel: w152 -> [w216 w224]
                      tunnel: w142 -> [_ w221]
                      tunnel: [w216 w220] -> w125
                      tunnel: w130 -> [_ w223]
                      tunnel: w129 -> [_ w222]
                      frame False {
                        # "不插入"
                      }
                      frame True {
                        # "尾插入 两点"
                        n91 = Insert Into Array(array=w224, new element #1=w222, new element #2=w221) -> (w220:timestamp[])  [unwired: 1 in]
                        n92 = Insert Into Array(array=w225, new element #1=w223, new element #2=w218) -> (w219:dbl[])  [unwired: 1 in]
                      }
                    }
                    n93 = case shown="真" w134 {
                      tunnel: [w234 w238] -> w171
                      tunnel: w121 -> [w234 w242]
                      tunnel: w161 -> [_ w235]
                      tunnel: w142 -> [_ w236]
                      tunnel: w170 -> [w233 w241]
                      tunnel: [w233 w237] -> w127
                      tunnel: w131 -> [_ w240]
                      tunnel: w129 -> [_ w239]
                      frame False {
                        # "不插入"
                      }
                      frame True {
                        # "尾插入 两点"
                        n94 = Insert Into Array(array=w242, new element #1=w240, new element #2=w235) -> (w238:dbl[])  [unwired: 1 in]
                        n95 = Insert Into Array(array=w241, new element #1=w239, new element #2=w236) -> (w237:timestamp[])  [unwired: 1 in]
                      }
                    }
                    n96 = Index Array(array=w125) -> (element=w124:timestamp)  [unwired: 1 in]
                    n97 = Index Array(array=w127) -> (element=w126:timestamp)  [unwired: 1 in]
                    n98 = Less? "过时？"(x=w124, y=w139) -> (x < y?=w151:bool)
                    n99 = Less? "过时？"(x=w126, y=w139) -> (x < y?=w169:bool)
                    n100 = Or(x=w119, y=w169) -> (x .or. y?=w123:bool)
                    n101 = Or(x=w118, y=w151) -> (x .or. y?=w122:bool)
                    n102 = case shown="真" w122 {
                      tunnel: w128 -> [w210 w214]
                      tunnel: w125 -> [w209 w213]
                      tunnel: 0 ("索引") -> [_ w215]
                      tunnel: [w210 w212] -> w117
                      tunnel: [w209 w211] -> w156
                      frame False {
                      }
                      frame True {
                        # "头删除"
                        n103 = Delete From Array(array=w214, index=w215) -> (array with subset deleted=w212:dbl[])  [unwired: 1 in, 1 out]
                        n104 = Delete From Array(array=w213, index=w215) -> (array with subset deleted=w211:timestamp[])  [unwired: 1 in, 1 out]
                      }
                    }
                    n105 = case shown="真" w123 {
                      tunnel: w171 -> [w227 w232]
                      tunnel: w127 -> [w226 w230]
                      tunnel: 0 ("索引") -> [_ w231]
                      tunnel: [w227 w229] -> w116
                      tunnel: [w226 w228] -> w140
                      frame False {
                      }
                      frame True {
                        # "头删除"
                        n106 = Delete From Array(array=w232, index=w231) -> (array with subset deleted=w229:dbl[])  [unwired: 1 in, 1 out]
                        n107 = Delete From Array(array=w230, index=w231) -> (array with subset deleted=w228:timestamp[])  [unwired: 1 in, 1 out]
                      }
                    }
                    n108 = Array Size(array=w116) -> (size(s)=w173:i32)
                    n109 = Array Size(array=w117) -> (size(s)=w155:i32)
                    n110 = Array Max & Min "最小限值2"(array=w117) -> (min value=w111:dbl)  [unwired: 3 out]
                    n111 = Array Max & Min "最大限值1"(array=w116) -> (max value=w114:dbl, min value=w113:dbl)  [unwired: 2 out]
                    n112 = Decrement(x=w173) -> (x-1=w174:i32)
                    n113 = Decrement(x=w155) -> (x-1=w154:i32)
                    n114 = Index Array(array=w116, index #2=w174) -> (element #1=w138:dbl, element #2=w137:dbl)  [unwired: 1 in]
                    n115 = Index Array(array=w117, index #2=w154) -> (element #1=w157:dbl, element #2=w158:dbl)  [unwired: 1 in]
                    n116 = Array Max & Min(array=w188) -> (max value=w179:dbl, min value=w178:dbl)  [unwired: 2 out]
                    n117 = Build Array (concatenate)(w138, w116, w137) -> (w136:dbl[])
                    n118 = Build Array (concatenate)(w139, w140, w129) -> (w135:timestamp[])
                    n119 = Build Array (concatenate)(w157, w117, w158) -> (w160:dbl[])
                    n120 = Build Array (concatenate)(w139, w156, w129) -> (w159:timestamp[])
                    n121 = Not Equal?(x=inf, y=w161) -> (x != y?=w176:bool)
                    n122 = case shown="真" w176 {
                      tunnel: w179 -> [w244 w250]
                      tunnel: [w244 w249] -> w112
                      tunnel: w113 -> [_ w248]
                      tunnel: w178 -> [w243 w247]
                      tunnel: [w243 w246] -> w177
                      tunnel: w114 -> [_ w245]
                      frame False {
                        # "报警限值 Inf 无效"
                      }
                      frame True {
                        # "报警限值有效"
                        n123 = Max & Min(x=w250, y=w245) -> (max(x,y)=w249:dbl)  [unwired: 1 out]
                        n124 = Max & Min(x=w247, y=w248) -> (min(x,y)=w246:dbl)  [unwired: 1 out]
                      }
                    }
                    n125 = Bundle(w135, w136) -> (w195:cluster{timestamp[], dbl[]})  [unwired: 1 in]
                    n126 = Bundle(w159, w160) -> (w141:cluster{timestamp[], dbl[]})  [unwired: 1 in]
                    n127 = Greater?(x=w112, y=w111) -> (0:w110:bool)
                    n128 = Subtract(x=w112, y=w177) -> (x-y=w187:dbl)
                    n129 = Multiply(x=w187, y=0.1) -> (x*y=w184:dbl)
                    n130 = Subtract(x=w139, y=w208) -> (x-y=w206:dbl)
                    n131 = control-ref of="XY图"() -> (w108:refnum<vi>)
                    n132 = Subtract(x=w129, y=w208) -> (x-y=w207:dbl)
                    n133 = Add(x=w112, y=w184) -> (x+y=w185:dbl)
                    n134 = Subtract(x=w177, y=w184) -> (x-y=w180:dbl)
                    n135 = Less Or Equal To 0?(x=w180) -> (x <= 0?=w183:bool)
                    n136 = property on="属性节点" class="XY图 (严格)"(reference=w108, "Active Plot"=w194, "Plot.Visible?"=w110) -> (reference out=w107:refnum<vi>, error out=w189:errorcluster)  [unwired: 1 in]
                    n137 = Select(t=0.0, s=w183, f=w180) -> (s? t:f=w181:dbl)
                    n138 = property on="属性节点" class="XY图 (严格)"(reference=w107, error in=w189, "XScale.Maximum"=w207, "XScale.Minimum"=w206, "YScale.Maximum"=w185, "YScale.Minimum"=w181) -> ()  [unwired: 2 out]
                    n139 = in-place-match #2(w109) -> (w99:cluster{timestamp[], dbl[]})
                    n140 = in-place-match #3(w195) -> (w101:cluster{timestamp[], dbl[]})
                    n141 = in-place-match #4(w141) -> (w100:cluster{timestamp[], dbl[]})
                  }
                  n142 = in-place-array #1(w99, w101, w100) -> (w91:cluster{timestamp[], dbl[]}[])  [unwired: 3 out]
                }
                n143 = property on="坐标映射信号" class="Bool (严格)"("Val(Sgnl)"=w89) -> ()  [unwired: 2 in, 2 out]
                n144 = local write "XY图"(w91) -> ()
              }
            }
            n145 = Unbundle By Name(w78) -> ("限值1"=w54:dbl, "限值2"=w52:dbl, "探头限值"=w55:T7)
            n146 = Unbundle By Name(w44) -> ("数值"=w84:dbl)
            n147 = Index Array(array="报警方式[]", index=w64) -> (element=w69:string)
            n148 = Equal?(x=w55, y=w66) -> (x = y?=w68:bool)
            n149 = Less Than 0?(x=w84) -> (x < 0?=w83:bool)
            n150 = case shown="真" w76 {
              tunnel: w83 -> [_ _]
              tunnel: w84 -> [_ w268]
              tunnel: [_ w267] -> w81
              tunnel: [_ w266] -> w82
              tunnel: [enum16{"正常", "未启用", "离线", "一级报警", "二级报警"}."未启用" ("探头状态") w265] -> w80
              tunnel: w75 -> [_ w264]
              frame False {
                # "未启用的探头"
              }
              frame True {
                w262 = 1000.0 ("y")
                # "启用的探头"
                n151 = case shown="\"累积报警\"" w264 {
                  tunnel: [探头状态."正常" ("探头状态") 探头状态."一级报警" ("探头状态") 探头状态."二级报警" ("探头状态") 探头状态."离线" ("探头状态") 探头状态."禁用" ("探头状态") 探头状态."累积报警" ("探头状态")] -> w265
                  frame "正常", Default {
                  }
                  frame "一级报警" {
                  }
                  frame "二级报警" {
                  }
                  frame "离线" {
                  }
                  frame "禁用" {
                  }
                  frame "累积报警" {
                  }
                }
                n152 = Greater Or Equal?(x=w268, y=w262) -> (x >= y?=w263:bool)
                n153 = case shown="真" w263 {
                  tunnel: w268 -> [w276 w280]
                  tunnel: w262 -> [_ w279]
                  tunnel: [w276 w278] -> w267
                  tunnel: [enum16{"μ", "m"}."μ" ("单位") enum16{"μ", "m"}."m" ("单位")] -> w266
                  frame False {
                  }
                  frame True {
                    n154 = Divide(x=w280, y=w279) -> (x/y=w278:dbl)
                  }
                }
              }
            }
            "测量值" <- w81
            "单位" <- w82
            n155 = Select(t=w70, s=w68, f=w67) -> (s? t:f=w58:string)
            n156 = Select(t=w70, s=w68, f=w69) -> (s? t:f=w56:string)
            n157 = Select(t=w67, s=w68, f=w70) -> (s? t:f=w59:string)
            n158 = Select(t=w69, s=w68, f=w70) -> (s? t:f=w57:string)
            n159 = call "带单位测量值字符串.vi"("测量值"=w52) -> ("结果"=w51:string)  [unwired: 10 in]
            n160 = call "带单位测量值字符串.vi"("测量值"=w54) -> ("结果"=w53:string)  [unwired: 10 in]
            n161 = call "二级限值"("二级限值"=w51, "说明"=w58, "报警方式"=w56) -> ("Result"=→"限值2":string)  [unwired: 11 in, 1 out]
            n162 = call "一级限值"("一级限值"=w53, "说明"=w59, "报警方式"=w57) -> ("Result"=→"限值1":string)  [unwired: 11 in, 1 out]
            n163 = property on="探头状态" class="Enum (严格)"("Val(Sgnl)"=w80) -> ()  [unwired: 2 in, 2 out]
            n164 = Unbundle By Name(w63) -> ("探头地址与信息.累积剂量"=w50:dbl, "探头地址与信息.累积限值"=w49:dbl)
            n165 = call "带单位测量值字符串.vi"("测量值"=w49) -> ("结果"=w48:string)  [unwired: 10 in]
            n166 = call "带单位测量值字符串.vi"("精度(2)"=i16 3 ("精度(6)"), "测量值"=w50) -> ("结果"=w47:string)  [unwired: 9 in]
            n167 = call "累积/限值"("累积剂量"=w47, "累积限值"=w48) -> ("Result"=→"累积":string)  [unwired: 12 in, 1 out]
          }
          event "XY图": Mouse Enter {
            # "显示悬浮数组"
            n168 = event-data() -> ()  [unwired: 1 in, 4 out]
            n169 = property on="数值" class="Str"("Visible"=TRUE ("可见")) -> ()  [unwired: 2 in, 2 out]
          }
          event "XY图": Mouse Leave {
            # "隐藏悬浮数值"
            n170 = event-data() -> ()  [unwired: 1 in, 4 out]
            n171 = property on="数值" class="Str"("Visible"=FALSE ("可见")) -> ()  [unwired: 2 in, 2 out]
          }
          event "XY图": Mouse Move {
            # "触发 数值映射事件"
            n172 = event-data() -> ("Coords"=w286:T4)  [unwired: 1 in, 4 out]
            n173 = flat-sequence {
              tunnel: w286 -> [w287]
              frame #0 {
                n174 = local write "鼠标坐标"(w287) -> ()
              }
              frame #1 {
                n175 = property on="坐标映射信号" class="Bool (严格)"("Val(Sgnl)"=TRUE ("值(信号)")) -> ()  [unwired: 2 in, 2 out]
                n176 = Wait (ms)(milliseconds to wait=u32 10 ("等待时间（毫秒）")) -> ()  [unwired: 1 out]
              }
            }
          }
          event "坐标映射信号": Value Change {
            # "数值映射"
            n177 = event-data() -> ()  [unwired: 1 in, 6 out]
            n178 = stacked-sequence {
              tunnel: [w302] -> w294
              frame #0 {
                n179 = Get Date/Time In Seconds() -> (seconds since 1Jan1904=w302:timestamp)
              }
            }
            n180 = Unbundle(w290) -> (w291:timestamp[], w292:dbl[])
            n181 = property on="数值" class="Str"() -> ("Visible"=w297:bool)  [unwired: 2 in, 2 out]
            n182 = Empty Array?(array=w292) -> (empty?=w293:bool)
            n183 = Not(x=w293) -> (.not. x?=w298:bool)
            n184 = And(x=w298, y=w297) -> (x .and. y?=w296:bool)
            n185 = case shown="真" w296 {
              tunnel: w291 -> [_ w324]
              tunnel: w292 -> [_ w323]
              tunnel: w294 -> [w303 w317]
              tunnel: [w303 w317] -> w295
              frame False {
                # "空数组，或悬浮数值不可见"
              }
              frame True {
                w334 = 1000.0 ("y")
                # "非空数组，且悬数值可见"
                n186 = control-ref of="XY图"() -> (w315:refnum<vi>)
                n187 = invoke on="调用节点" class="XY图 (严格)" method="Map Coords To XY"(reference=w315, "Coords"="鼠标坐标") -> ("XY"=w336:cluster{"X":dbl, "Y":dbl})  [unwired: 5 in, 6 out]
                n188 = Unbundle By Name("鼠标坐标") -> ("Horizontal"=w305:i32, "Vertical"=w304:i32)
                n189 = property on="数值" class="Str"() -> (error out=w319:errorcluster, "Bounds"=w318:T17)  [unwired: 2 in, 1 out]
                n190 = Unbundle By Name(w318) -> ("Width"=w309:u32, "Height"=w308:u32)
                n191 = Unbundle By Name(w336) -> ("X"=w329:dbl)
                n192 = Subtract(x=w324, y=timestamp(0 s since 1904-01-01)) -> (x-y=w327:dbl[])
                n193 = call "快速逼近索引法.vi"("数值"=w329, "数组"=w327) -> ("最近索引"=w326:i32)  [unwired: 9 in]
                n194 = Divide(x=w309, y=u32 2) -> (x/y=w311:dbl)
                n195 = Index Array(array=w323, index=w326) -> (element=w325:dbl)
                n196 = Subtract(x=w305, y=w311) -> (x-y=w307:dbl)
                n197 = Subtract(x=w304, y=w308) -> (x-y=w312:u32)
                n198 = Greater Or Equal?(x=w325, y=w334) -> (x >= y?=w335:bool)
                n199 = Subtract(x=w312, y=u32 10) -> (x-y=w306:u32)
                n200 = case shown="假" w335 {
                  tunnel: w325 -> [w338 w342]
                  tunnel: w334 -> [_ w341]
                  tunnel: [w338 w340] -> w332
                  tunnel: [" μSv/h" " mSv/h"] -> w330
                  frame False {
                    # "mSv/h"
                  }
                  frame True {
                    # "uSv/h"
                    n201 = Divide(x=w342, y=w341) -> (x/y=w340:dbl)
                  }
                }
                n202 = Bundle By Name(cluster=T14 {"Left"=0, "Top"=0} ("位置"), "Left"=w307, "Top"=w306) -> (w321:T14)
                n203 = property on="数值" class="Str"(error in=w319, "Position"=w321) -> ()  [unwired: 1 in, 2 out]
                n204 = Number To Fractional String(number=w332, precision (6)=i16 2 ("精度(6)")) -> (F-format string=w331:string)  [unwired: 2 in]
                n205 = Concatenate Strings(w331, w330) -> (→"数值":string)
                n206 = Wait (ms)(milliseconds to wait=u32 10 ("等待时间（毫秒）")) -> ()  [unwired: 1 out]
              }
            }
            n207 = stacked-sequence {
              tunnel: w295 -> [w300]
              frame #0 {
                # "净处理时间为\n最少 3μs\n300点满数组 5~20ms"
                n208 = Get Date/Time In Seconds() -> (seconds since 1Jan1904=w301:timestamp)
                n209 = Subtract(x=w301, y=w300) -> (x-y=→"计算时间":dbl)
              }
            }
          }
          event "探头状态": Value Change {
            n210 = event-data() -> ("OldVal"=w349:enum16{"正常", "离线", "禁用", "一级报警", "二级报警", "累积报警"}, "NewVal"=w350:enum16{"正常", "离线", "禁用", "一级报警", "二级报警", "累积报警"})  [unwired: 1 in, 4 out]
            n211 = control-ref of="窗格"() -> (w348:refnum<vi>)
            n212 = control-ref of="XY图"() -> (w347:refnum<vi>)
            n213 = case shown="\"正常\", 默认" w350 {
              tunnel: w349 -> [w354 _ w369 _ _]
              tunnel: w348 -> [w353 _ w368 _ _]
              tunnel: w347 -> [w352 _ w367 _ _]
              tunnel: [_ _ _ _ TRUE] -> w344
              tunnel: [_ _ _ TRUE _] -> w343
              frame "正常", Default {
                # "从禁用到正常 需改变禁用状态"
                n214 = case shown="\"禁用\"" w354 {
                  tunnel: w353 -> [_ w360]
                  tunnel: w352 -> [_ w359]
                  frame "正常", Default {
                  }
                  frame "禁用" {
                    w358 = T18."Disabled" ("禁用")
                    # "原值是禁用，现在改变状态"
                    n215 = property class="Pane"(reference=w360) -> ("Controls[]"=w361:refnum<vi>[])  [unwired: 1 in, 2 out]
                    n216 = Initialize Array(cluster{timestamp[], dbl[]} {[], []}, 3 ("维数大小")) -> (w355:cluster{timestamp[], dbl[]}[])
                    n217 = for {
                      tunnel: w361 -> [w363] mode=indexing
                      workers-P: _ -> [_]
                      tunnel: w358 -> [w362]
                      # "改变禁用效果"
                      n218 = property class="Ctl"(reference=w363, "DisabledEnum"=w362) -> ()  [unwired: 1 in, 2 out]
                    }
                    n219 = property class="XYGraph (严格)"(reference=w359, "DisabledEnum"=w358, "Value"=w355) -> ()  [unwired: 1 in, 2 out]
                  }
                }
              }
              frame "离线" {
                # "无需动作"
                n220 = Initialize Array(cluster{timestamp[], dbl[]} {[], []}, 3 ("维数大小")) -> (w364:cluster{timestamp[], dbl[]}[])
                n221 = local write "XY图"(w364) -> ()
              }
              frame "禁用" {
                # "从非禁用到禁用需改变禁用状态"
                n222 = case shown="\"正常\", 默认" w369 {
                  tunnel: w368 -> [w372 _]
                  tunnel: w367 -> [w370 _]
                  frame "正常", Default {
                    w371 = T18."Disabled and Grayed Out" ("禁用")
                    # "原值是 非禁用状态，现在改变为禁用变灰"
                    n223 = property class="Pane"(reference=w372) -> ("Controls[]"=w373:refnum<vi>[])  [unwired: 1 in, 2 out]
                    n224 = for {
                      tunnel: w373 -> [w375] mode=indexing
                      workers-P: _ -> [_]
                      tunnel: w371 -> [w374]
                      # "改变禁用效果"
                      n225 = property class="Ctl"(reference=w375, "DisabledEnum"=w374) -> ()  [unwired: 1 in, 2 out]
                    }
                    n226 = property class="XYGraph (严格)"(reference=w370, "DisabledEnum"=w371) -> ()  [unwired: 1 in, 2 out]
                  }
                  frame "禁用" {
                    # "原来就是禁用状态，不改变"
                  }
                }
              }
              frame "一级报警", "二级报警" {
                # "闪烁"
              }
              frame "累积报警" {
              }
            }
            n227 = control-ref of="测量值"() -> (w345:refnum<vi>)
            n228 = control-ref of="累积"() -> (w346:refnum<vi>)
            n229 = property class="DigNum (严格)"(reference=w345, "Blinking"=w343) -> ()  [unwired: 1 in, 2 out]
            n230 = property class="Str"(reference=w346, "Blinking"=w344) -> ()  [unwired: 1 in, 2 out]
          }
          event Pane Size {
            w398 = cluster{"所在窗格高度":u32, "字号":u32} {"所在窗格高度"=0, "字号"=0}  # 原始尺寸
            # "左窗格大小改变，要改变字号"
            n231 = event-data() -> ("NewBnds"=w405:T19)  [unwired: 1 in, 5 out]
            n232 = local read "初始尺寸"() -> (w409:T1)
            n233 = Unbundle By Name(w405) -> ("Bottom"=w406:i16, "Top"=w407:i16)
            n234 = Subtract(x=w406, y=w407) -> (x-y=w395:i16)
            n235 = Unbundle By Name(w409) -> ("边界:区域高度"=w396:u32, "最大字号"=w408:T13)
            n236 = Unbundle By Name(w408) -> ("限值信息"=w394:u32, "测量值"=w393:u32, "序号"=w392:u32, "名称"=w391:u32, "单位"=w390:u32, "状态"=w389:u32, "悬浮框"=w385:u32)
            n237 = Bundle By Name(cluster=w398, "所在窗格高度"=w396) -> (w386:cluster{"所在窗格高度":u32, "字号":u32})
            n238 = Bundle By Name(cluster=T15 {"原始尺寸"={"所在窗格高度"=0, "字号"=0}, "new所在窗格高度"=0} ("输出簇"), "new所在窗格高度"=w395) -> (w387:T15)
            n239 = Bundle By Name(cluster=w386, "字号"=w392) -> (w401:cluster{"所在窗格高度":u32, "字号":u32})
            n240 = Bundle By Name(cluster=w386, "字号"=w391) -> (w402:cluster{"所在窗格高度":u32, "字号":u32})
            n241 = Bundle By Name(cluster=w386, "字号"=w390) -> (w403:cluster{"所在窗格高度":u32, "字号":u32})
            n242 = Bundle By Name(cluster=w386, "字号"=w385) -> (w388:cluster{"所在窗格高度":u32, "字号":u32})
            n243 = Bundle By Name(cluster=w386, "字号"=w389) -> (w404:cluster{"所在窗格高度":u32, "字号":u32})
            n244 = Bundle By Name(cluster=w386, "字号"=w393) -> (w400:cluster{"所在窗格高度":u32, "字号":u32})
            n245 = Bundle By Name(cluster=w386, "字号"=w394) -> (w399:cluster{"所在窗格高度":u32, "字号":u32})
            n246 = Bundle By Name(cluster=w387, "原始尺寸"=w399) -> (w384:T15)
            n247 = Bundle By Name(cluster=w387, "原始尺寸"=w400) -> (w383:T15)
            n248 = Bundle By Name(cluster=w387, "原始尺寸"=w401) -> (w382:T15)
            n249 = Bundle By Name(cluster=w387, "原始尺寸"=w402) -> (w381:T15)
            n250 = Bundle By Name(cluster=w387, "原始尺寸"=w403) -> (w380:T15)
            n251 = Bundle By Name(cluster=w387, "原始尺寸"=w388) -> (w378:T15)
            n252 = Bundle By Name(cluster=w387, "原始尺寸"=w404) -> (w379:T15)
            n253 = control-ref of="累积"() -> (w418:refnum<vi>)
            n254 = control-ref of="限值1"() -> (w420:refnum<vi>)
            n255 = control-ref of="限值2"() -> (w419:refnum<vi>)
            n256 = control-ref of="XY图"() -> (w415:refnum<vi>)
            n257 = control-ref of="探头信息"() -> (w417:refnum<vi>)
            n258 = control-ref of="数值"() -> (w414:refnum<vi>)
            n259 = control-ref of="单位"() -> (w412:refnum<vi>)
            n260 = control-ref of="探头状态"() -> (w411:refnum<vi>)
            n261 = control-ref of="探头地址"() -> (w410:refnum<vi>)
            n262 = control-ref of="测量值"() -> (w413:refnum<vi>)
            n263 = call "字符串控件字号自适应.vi"("新旧尺寸信息"=w378, "字符串控件-引用"=w414) -> ()  [unwired: 8 in, 2 out]
            n264 = call "枚举控件字号自适应.vi"("新旧尺寸信息"=w379, "枚举控件-引用"=w411) -> ()  [unwired: 8 in, 2 out]
            n265 = call "字符串控件字号自适应.vi"("新旧尺寸信息"=w384, "字符串控件-引用"=w420) -> ("字号"=w416:u32)  [unwired: 8 in, 1 out]
            n266 = call "字符串控件字号自适应.vi"("新旧尺寸信息"=w384, "字符串控件-引用"=w419) -> ()  [unwired: 8 in, 2 out]
            n267 = call "字符串控件字号自适应.vi"("新旧尺寸信息"=w384, "字符串控件-引用"=w418) -> ()  [unwired: 8 in, 2 out]
            n268 = call "枚举控件字号自适应.vi"("新旧尺寸信息"=w380, "枚举控件-引用"=w412) -> ()  [unwired: 8 in, 2 out]
            n269 = call "字符串控件字号自适应.vi"("新旧尺寸信息"=w381, "字符串控件-引用"=w417) -> ()  [unwired: 8 in, 2 out]
            n270 = call "数值控件字号自适应.vi"("新旧尺寸信息"=w383, "数值控件-引用"=w413) -> ()  [unwired: 8 in, 2 out]
            n271 = call "枚举控件字号自适应.vi"("新旧尺寸信息"=w382, "枚举控件-引用"=w410) -> ()  [unwired: 8 in, 2 out]
            n272 = Decrement(x=w416) -> (x-1=w421:u32)
            n273 = call "XY图标尺字号自适应.vi"("标尺字号"=w421, "XY图-引用"=w415) -> ()  [unwired: 9 in, 1 out]
          }
        }
      }
    }
  }
